vi "Read_Value_Arduino.vi"(0 "VISA resource name":refnum<visa-resource-name>, 1 "write buffer":string, 2 "format string (%.;%f)":string="%.;%f", 3 "error in (no error)":errorcluster) -> (4 "output":dbl, 5 "VISA resource name out":refnum<visa-resource-name>, 6 "concatenated string":string, 7 "error out":errorcluster)   [LabVIEW 2018]
panel:
  out "code":i32
  out "source":string
  out "status":bool
  out "Serial Settings:Number of Bytes at Serial Port":u32
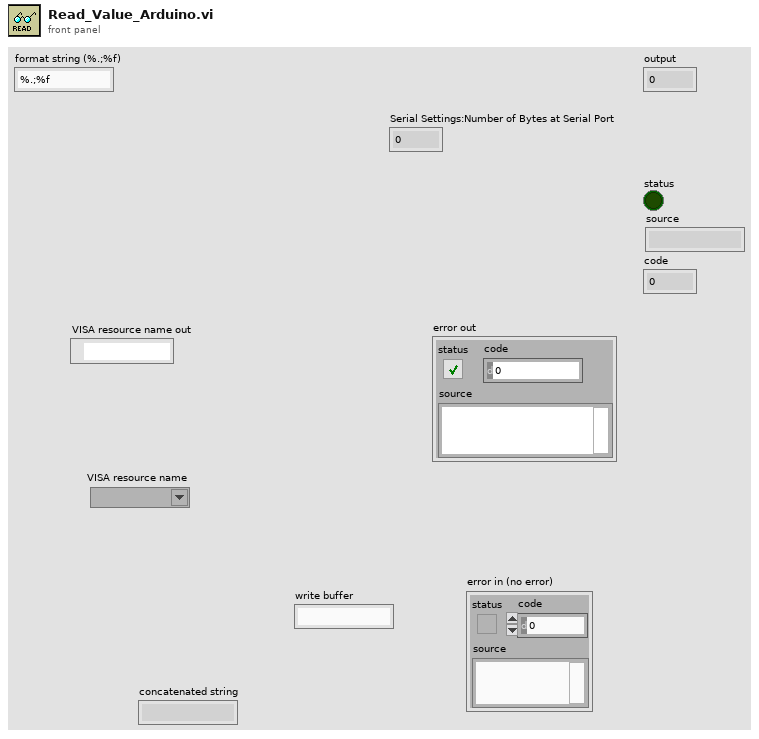
[diagram p1: front panel]
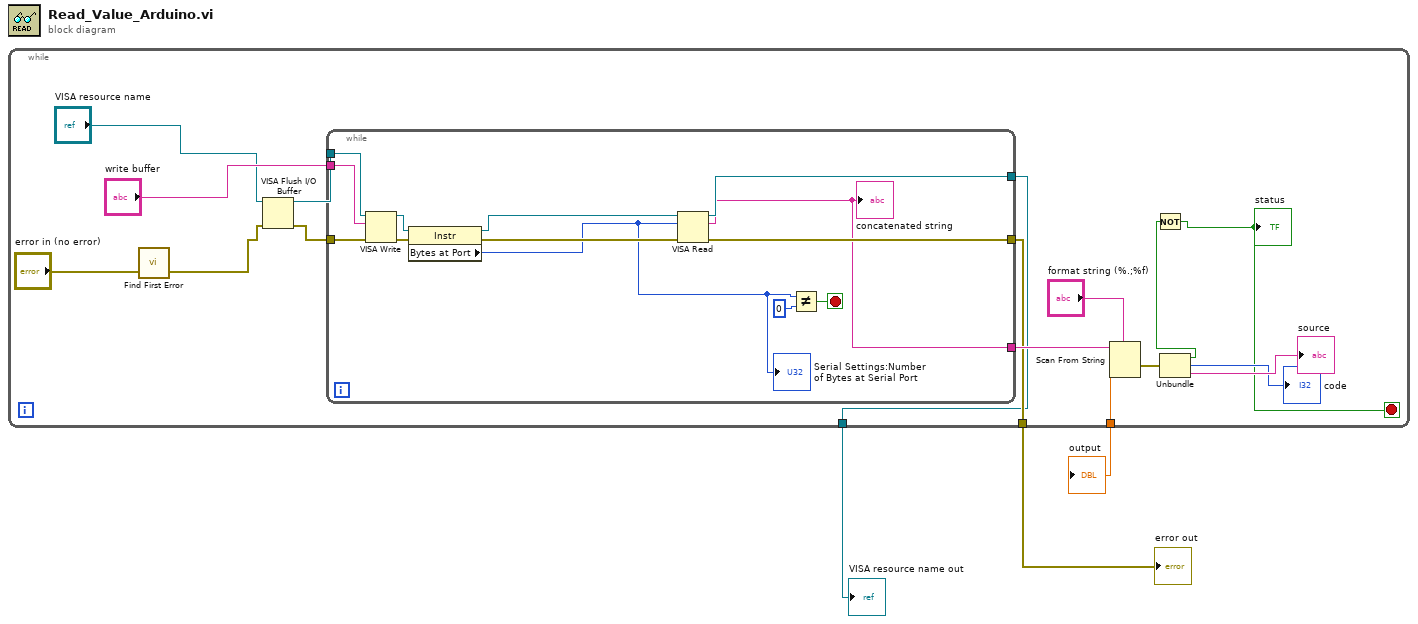
[diagram p0: block diagram]
diagram:
  n1 = while {
    tunnel: [w11] -> w3
    tunnel: [w9] -> w2
    tunnel: [w8] -> w1
    stop <- w4 stop-if-true
    n2 = call <vilib>:"Find First Error.vi"("error in (no error)"="error in (no error)") -> ("error out"=w15:errorcluster)  [unwired: 3 in, 1 out]
    n3 = VISA Flush I/O Buffer(VISA resource name="VISA resource name", error in (no error)=w15) -> (VISA resource name out=w16:refnum<visa-resource-name>, error out=w14:errorcluster)  [unwired: 1 in]
    n4 = while {
      tunnel: w16 -> [w26]
      tunnel: "write buffer" -> [w27]
      tunnel: w14 -> [w28]
      tunnel: [w25] -> w9
      tunnel: [w24] -> w8
      tunnel: [w20] -> w13
      stop <- w31 stop-if-true
      n5 = VISA Write(VISA resource name=w26, write buffer=w27, error in (no error)=w28) -> (VISA resource name out=w29:refnum<visa-resource-name>, error out=w30:errorcluster)  [unwired: 1 out]
      n6 = property class="Instr"(reference=w29, error in=w30) -> (reference out=w23:refnum<visa-resource-name>, error out=w22:errorcluster, "Bytes at Port"=w21:u32)
      "Serial Settings:Number of Bytes at Serial Port" <- w21
      n7 = VISA Read(VISA resource name=w23, byte count=w21, error in (no error)=w22) -> (VISA resource name out=w24:refnum<visa-resource-name>, read buffer=w20:string, error out=w25:errorcluster)  [unwired: 1 out]
      "concatenated string" <- w20
      n8 = Not Equal?(x=w21, y=0) -> (x != y?=w31:bool)
    }
    n9 = Scan From String(format string="format string (%.;%f)", input string=w13) -> (error out=w10:errorcluster, output 1=w11:dbl)  [unwired: 3 in, 2 out]
    n10 = Unbundle(w10) -> ("status"=w5:bool, "code"=→"code":i32, "source"=→"source":string)
    n11 = Not(x=w5) -> (.not. x?=w4:bool)
    "status" <- w4
  }
  "output" <- w3
  "error out" <- w2
  "VISA resource name out" <- w1
